vi "Trigger TimerDRV.vi"(8 "error in (no error)":errorcluster, 11 "TimerDRV in":refnum<class "TimerDRV.lvclass">) -> (0 "error out":errorcluster, 3 "TimerDRV out":refnum<class "TimerDRV.lvclass">)   [LabVIEW 2019, in "TimingDRV Engine.lvlib" / "TimerDRV.lvclass"]
uses:
  TimerDRV.lvclass
  TimerDRV.lvclass/TimerDRV.ctl
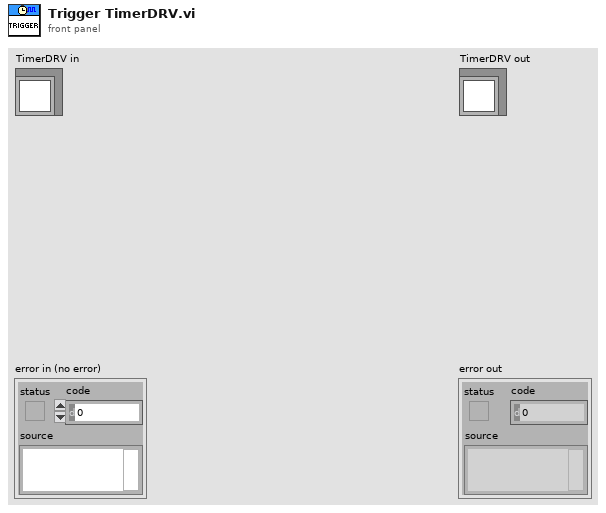
[diagram p1: front panel]
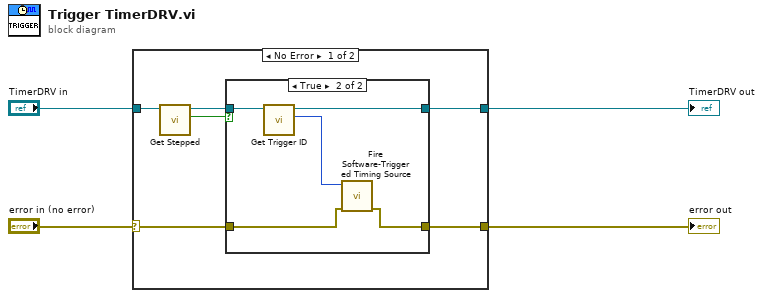
[diagram p0: block diagram]
diagram:
  n1 = case shown="No Error" "error in (no error)" {
    selector: "error in (no error)" -> [w9 w19]
    tunnel: [w8 w19] -> w3
    tunnel: [w10 w18] -> w1
    tunnel: "TimerDRV in" -> [w7 w18]
    frame No Error {
      n2 = call "Get Stepped.vi"("TimerDRV in"=w7) -> ("Stepped"=w5:bool, "TimerDRV out"=w6:refnum<class "TimerDRV.lvclass">)  [unwired: 9 in]
      n3 = case shown="True" w5 {
        tunnel: [w12 w16] -> w10
        tunnel: w9 -> [w11 w15]
        tunnel: [w11 w14] -> w8
        tunnel: w6 -> [w12 w13]
        frame False {
        }
        frame True {
          n4 = call "Get Trigger ID.vi"("TimerDRV in"=w13) -> ("Trigger ID"=w17:u8, "TimerDRV out"=w16:refnum<class "TimerDRV.lvclass">)  [unwired: 9 in]
          n5 = call <vilib>:"Fire Software-Triggered Timing Source.vi"("error in (no error)"=w15, "trigger ID"=w17) -> ("error out"=w14:errorcluster)  [unwired: 8 in, 1 out]
        }
      }
    }
    frame Error {
    }
  }
  "error out" <- w3
  "TimerDRV out" <- w1
